vi "DataBinding-receiver.vi"() -> ()   [LabVIEW 2020]
panel:
  in  "reveived item":dbl
  in  "stop":bool
  out "Waveform Chart":dbl(graph)
  out "Gauge":dbl(knob) scale=0.0..100.0
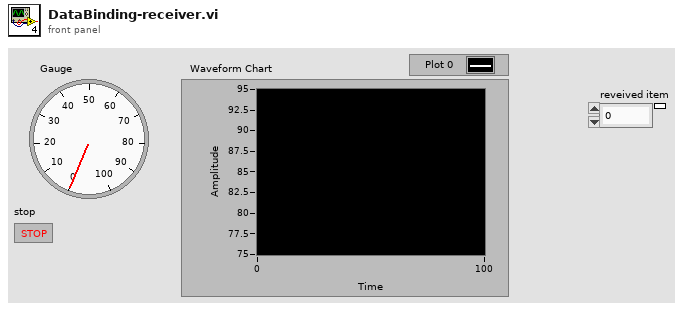
[diagram p1: front panel]
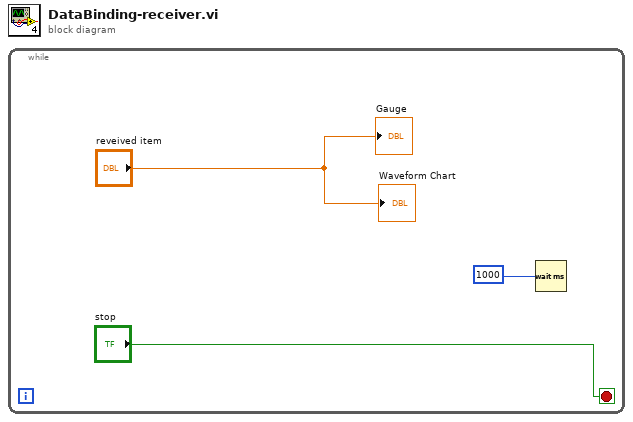
[diagram p0: block diagram]
diagram:
  n1 = while {
    stop <- "stop" stop-if-true
    n2 = Wait (ms)(milliseconds to wait=1000) -> ()  [unwired: 1 out]
    "Gauge" <- "reveived item"
    "Waveform Chart" <- "reveived item"
  }
